vi "playing with images.vi"() -> ()   [LabVIEW 2018]
panel:
  in  "Numeric":dbl
  in  "Numeric 2":dbl
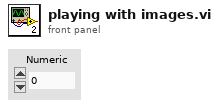
[diagram p1: front panel]
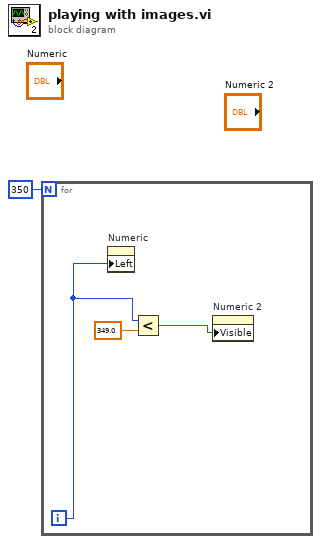
[diagram p0: block diagram]
diagram:
  n1 = for {
    N: 350 -> [_]
    i -> [w3]
    n2 = property on="Numeric" class="DigNum (strict)"("Left"=w3) -> ()  [unwired: 2 in, 2 out]
    n3 = Less?(x=w3, y=349.0) -> (x < y?=w2:bool)
    n4 = property on="Numeric 2" class="DigNum (strict)"("Visible"=w2) -> ()  [unwired: 2 in, 2 out]
  }
